vi "PV ActiveLine - CalibrationFactor (TPG361).vi"(7 "W/R":bool, 8 "Fehler (Eingang)":errorcluster, 10 "Set Calibration factor1":dbl=1.0 min=0.1 max=9.999 step=0.001 format="%.3f", 11 "Referenz in":refnum<visa-resource-name>) -> (0 "Cluster (Ausgang)":errorcluster, 2 "Get Calibration factor 1":dbl=0.000753 format="%.3f", 3 "Referenz out":refnum<visa-resource-name>)   [LabVIEW 2013, in "PV ActiveLine.lvlib"]
doc: "COR - Correction Factor\n\nCOR corresponds to the CAL command\n\nTransmit: COR [,a.aaa]\nReceive: a.aaa\n\na.aaa = Correction factor gauge 1"
uses:
  C:/Program Files (x86)/National Instruments/LabVIEW 2013/PV ActiveLine/PV ActiveLine.lvlib
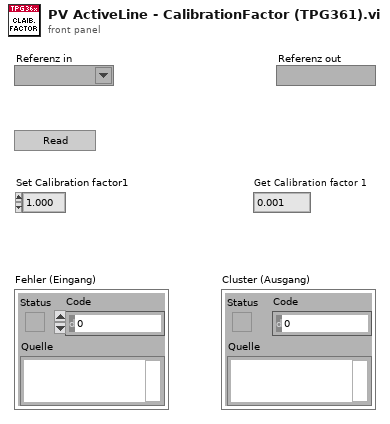
[diagram p1: front panel]
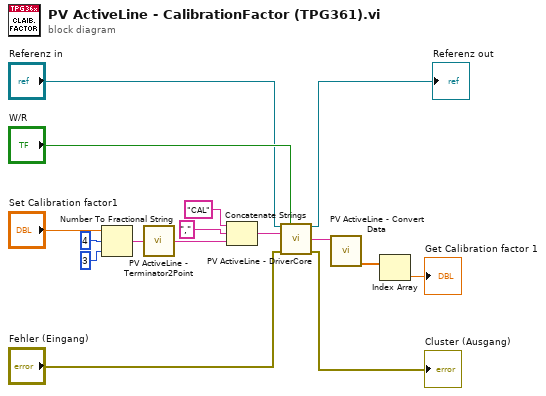
[diagram p0: block diagram]
diagram:
  n1 = Number To Fractional String(number="Set Calibration factor1", width (-)=i16 4, precision (6)=i16 3 ("width (-)")) -> (F-format string=w11:string)  [unwired: 1 in]
  n2 = call "PV ActiveLine - Terminator2Point.vi"("Eingangstring"=w11) -> ("Ausgangstring"=w10:string)
  n3 = Concatenate Strings("CAL", ",", w10) -> (w4:string)
  n4 = call "PV ActiveLine - DriverCore.vi"("Referenz in"="Referenz in", "Write/Read"="W/R", "Command"=w4, "Fehler (Eingang)"="Fehler (Eingang)") -> ("Referenz out"=→"Referenz out":refnum<visa-resource-name>, "String Out"=w3:string, "Cluster (Ausgang)"=→"Cluster (Ausgang)":errorcluster)  [unwired: 9 in]
  n5 = call "PV ActiveLine - Convert Data.vi"("String in"=w3) -> ("DBL out"=w2:dbl[])  [unwired: 7 in, 3 out]
  n6 = Index Array(array=w2) -> (element=→"Get Calibration factor 1":dbl)  [unwired: 1 in]
